vi "Write Output Data.vi"(10 "Output Data":T1, 11 "Logger in":refnum<class "TestDataLog.lvclass">) -> (3 "Logger out":refnum<class "TestDataLog.lvclass">)   [LabVIEW 2015, in "TestDataLog.lvclass"]
uses:
  TestDataLog.lvclass
  Typedefs/OutputData.ctl
  TestDataLog.lvclass/TestDataLog.ctl
  Typedefs/M1M3SSSTypedefs.lvlib
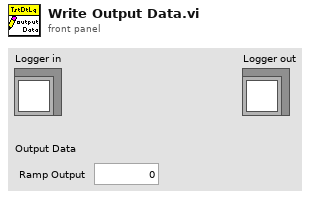
[diagram p1: front panel]
types:
  T1 = typedef "M1M3SSSTypedefs.lvlib/OutputData.ctl" = cluster{"Ramp Output":u16}
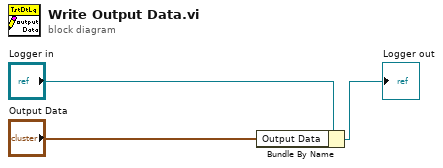
[diagram p0: block diagram]
diagram:
  n1 = Bundle By Name(cluster="Logger in", "Output Data"="Output Data") -> (→"Logger out":refnum<class "TestDataLog.lvclass">)
